vi "LabView360-6-Global-2.vi"() -> ()   [LabVIEW 2017]
uses:
  LabView360-6-Global.vi
panel:
  out "波形图表":dbl(graph)
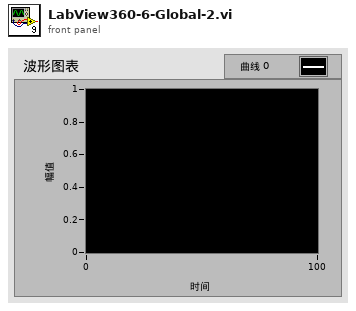
[diagram p1: front panel]
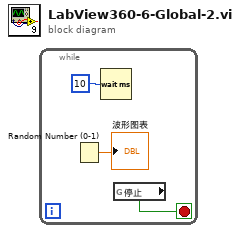
[diagram p0: block diagram]
diagram:
  n1 = while {
    stop <- w1 stop-if-true
    n2 = Random Number (0-1)() -> (number: 0 to 1=→"波形图表":dbl)
    n3 = Wait (ms)(milliseconds to wait=u32 10 ("等待时间（毫秒）")) -> ()  [unwired: 1 out]
    n4 = global read "LabView360-6-Global.vi" "停止"() -> (w1:bool)
  }
